vi "unused_getObjectRefs.vi"(6 "type(ClassName)":string="Wire", 8 "error in (no error)":errorcluster, 11 "BlockDiagram in":refnum<class "BlockDiagram.lvclass">) -> (0 "error out":errorcluster, 2 "refs":refnum<vi>[](array[refnum]), 3 "BlockDiagram out":refnum<class "BlockDiagram.lvclass">)   [LabVIEW 2023]
uses:
  BlockDiagram.lvclass/BlockDiagram.ctl
  <vilib>/Utility/traverseref.llb/TRef TravTarget.ctl
  BlockDiagram.lvclass
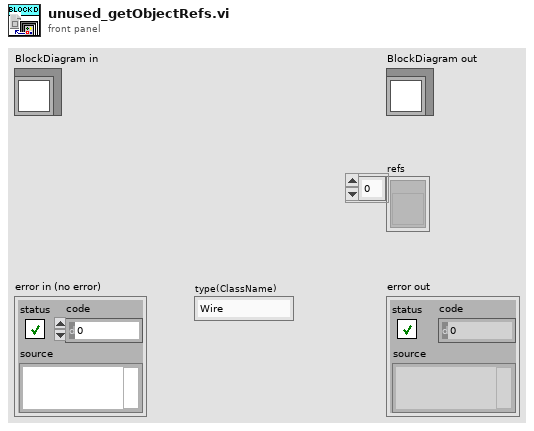
[diagram p1: front panel]
types:
  T1 = typedef "TRef TravTarget.ctl" = enum16{"FP", "BD", "Other"}
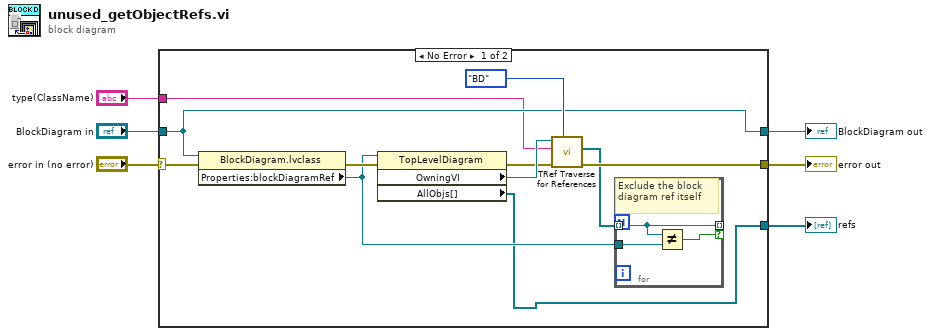
[diagram p0: block diagram]
diagram:
  n1 = case shown="No Error" "error in (no error)" {
    selector: "error in (no error)" -> [w12 w22]
    tunnel: [w10 w22] -> w5
    tunnel: [w14 w21] -> w3
    tunnel: "BlockDiagram in" -> [w14 w21]
    tunnel: "type(ClassName)" -> [w11 _]
    tunnel: [w7 _] -> w1
    frame No Error {
      n2 = property class="BlockDiagram.lvclass"(reference=w14, error in=w12) -> (error out=w13:errorcluster, "Properties:blockDiagramRef"=w9:refnum<vi>)  [unwired: 1 out]
      n3 = property on="Property Node" class="TopLevelDiagram"(reference=w9, error in=w13) -> (error out=w16:errorcluster, "OwningVI"=w17:refnum<vi>, "AllObjs[]"=w7:refnum<vi>[])  [unwired: 1 out]
      n4 = call <vilib>:"TRef Traverse for References.vi"("Traverse Target"=TRef_TravTarget."BD", "error in (no error)"=w16, "Class Name"=w11, "VI Refnum"=w17) -> ("error out"=w10:errorcluster, "References"=w8:refnum<vi>[])  [unwired: 1 in, 5 out]
      n5 = for {
        tunnel: w8 -> [w19] mode=indexing
        tunnel: w9 -> [w20]
        tunnel: [w19] -> _ mode=indexing if=w18
        # "Exclude the block diagram ref itself"
        n6 = Not Equal?(x=w19, y=w20) -> (x != y?=w18:bool)
      }
    }
    frame Error {
    }
  }
  "error out" <- w5
  "BlockDiagram out" <- w3
  "refs" <- w1
